vi "5_1.vi"() -> ()   [LabVIEW 2015]
panel:
  in  "Message 3":string
  in  "Message 2":string
  in  "Message 1":string
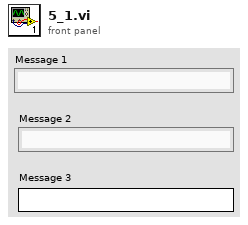
[diagram p1: front panel]
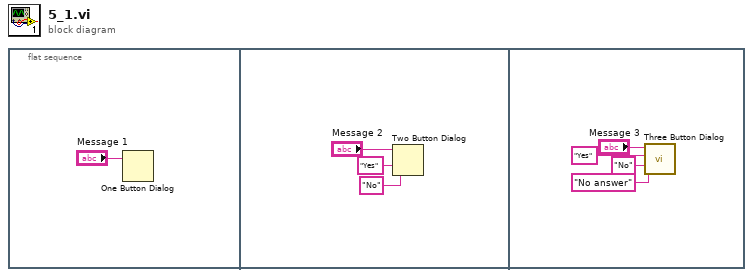
[diagram p0: block diagram]
diagram:
  n1 = flat-sequence {
    frame #0 {
      n2 = One Button Dialog(message="Message 1") -> ()  [unwired: 1 in, 1 out]
    }
    frame #1 {
      n3 = Two Button Dialog(message="Message 2", 1:"No" ("F button name (\"Cancel\")"), 2:"Yes" ("T button name (\"OK\")")) -> ()  [unwired: 1 out]
    }
    frame #2 {
      n4 = call <vilib>:"Three Button Dialog.vi"("Right Button Text (\"Cancel\")"="No answer" ("Right Button Text (\"Cancel\")"), "Center Button Text (\"No\")"="No" ("Center Button Text (\"No\")"), "Left Button Text (\"Yes\")"="Yes" ("Left Button Text (\"Yes\")"), "message"="Message 3") -> ()  [unwired: 7 in, 1 out]
    }
  }
